vi "Pre Launch Init.vi"(11 "定时循环控制器输入":refnum<class "Timed Loop Actor.lvclass">) -> (0 "error out":cluster{"状态":bool, "代码":i32, "源":string} caption="错误输出", 3 "定时循环控制器输出":refnum<class "Timed Loop Actor.lvclass">)   [LabVIEW 2015, in "Timed Loop Actor.lvlib" / "Timed Loop Actor.lvclass"]
uses:
  Timed Loop Actor.lvclass
  Timed Loop Actor.lvclass/Timed Loop Actor.ctl
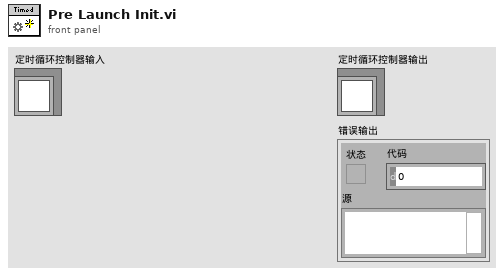
[diagram p1: front panel]
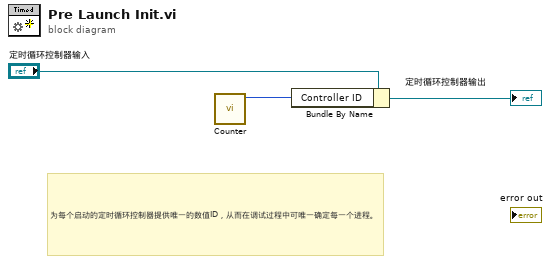
[diagram p0: block diagram]
diagram:
  # "为每个启动的定时循环控制器提供唯一的数值ID，从而在调试过程中可唯一确定每一个进程。"
  n1 = call "Counter.vi"() -> ("数值"=w1:u32)  [unwired: 11 in]
  n2 = Bundle By Name(cluster="定时循环控制器输入", "Controller ID"=w1) -> (→"定时循环控制器输出":refnum<class "Timed Loop Actor.lvclass">)
